vi "SetTriggerCount.vi"(8 "Error In":errorcluster, 10 "Count (1-3000)":u16, 11 "Keithley 6482 In":refnum<visa-resource-name>) -> (0 "Error Out":errorcluster, 3 "Keithley 6482 Out":refnum<visa-resource-name>)   [LabVIEW 8.6, in "Keithley-6482-Visa.lvlib"]
uses:
  Keithley-6482-Visa.lvlib
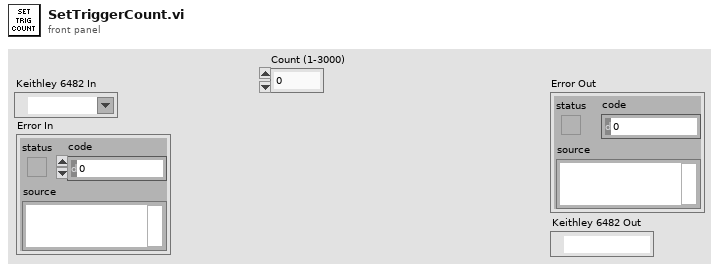
[diagram p1: front panel]
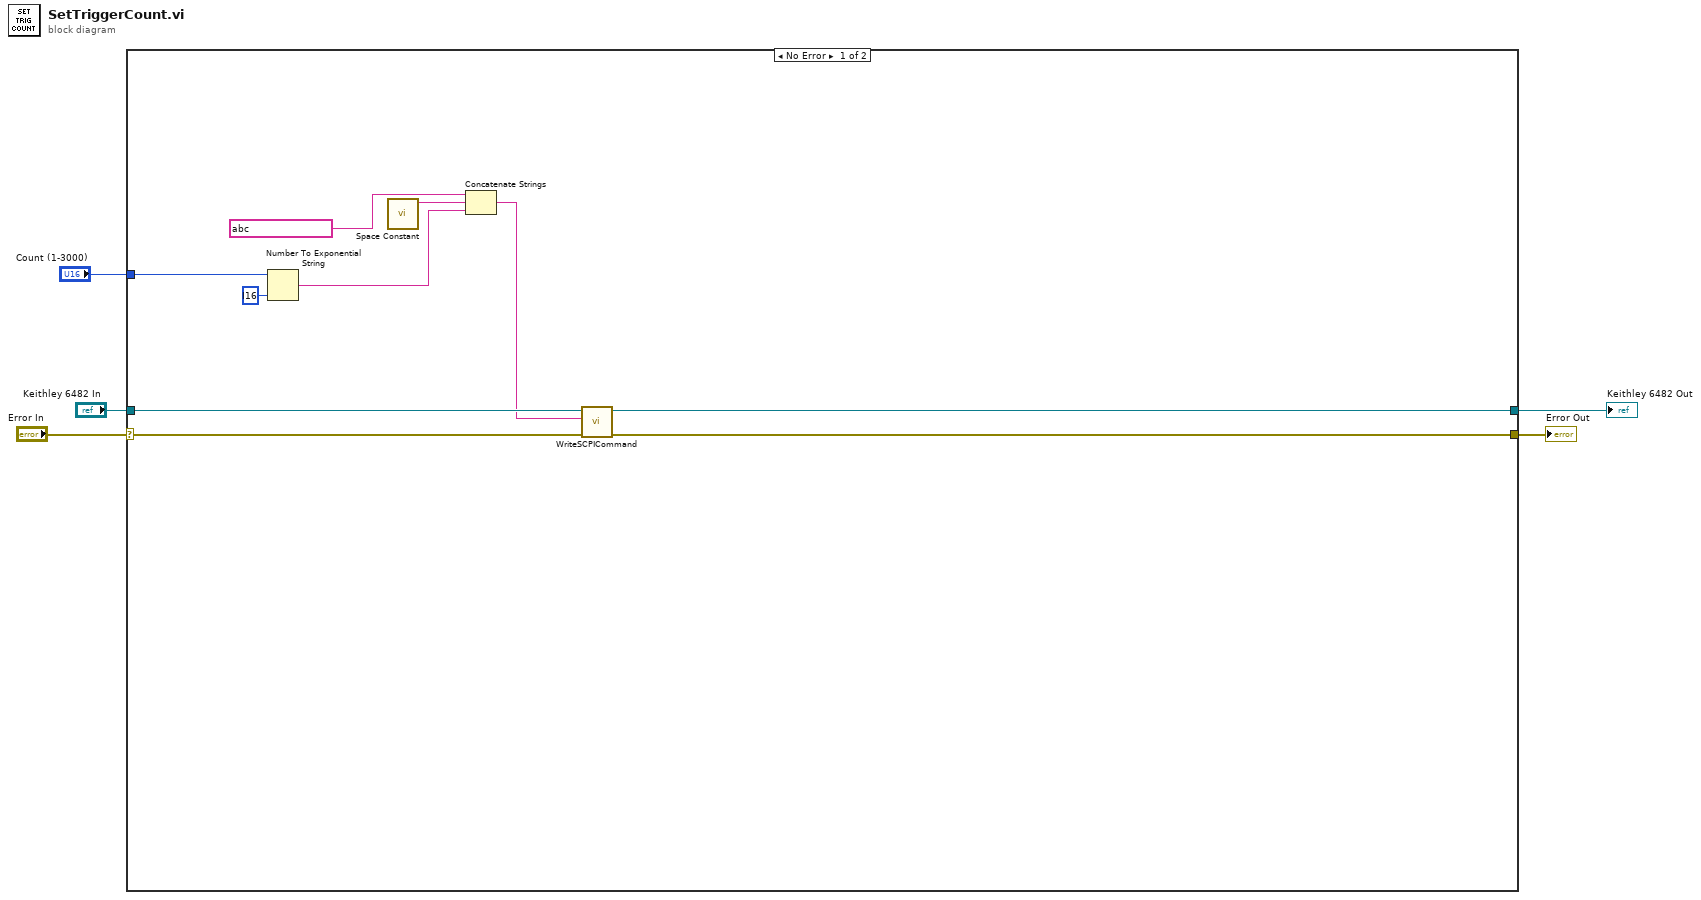
[diagram p0: block diagram]
diagram:
  n1 = case shown="No Error" "Error In" {
    selector: "Error In" -> [w15 w16]
    tunnel: "Keithley 6482 In" -> [w14 w17]
    tunnel: [w7 w16] -> w3
    tunnel: [w8 w17] -> w2
    tunnel: "Count (1-3000)" -> [w11 _]
    frame #0 {
      n2 = Number To Exponential String(number=w11, precision (6)=i16 ?) -> (E-format string=w10:string)  [unwired: 2 in]
      n3 = call <vilib>:"Space Constant.vi"() -> ("String"=w12:string)
      n4 = Concatenate Strings(string ? ("string"), w12, w10) -> (w9:string)
      n5 = call "WriteSCPICommand.vi"("Error In"=w15, "SCPI Command"=w9, "Keithley 6482 In"=w14) -> ("Error Out"=w7:errorcluster, "Keithley 6482 Out"=w8:refnum<visa-resource-name>)  [unwired: 7 in]
    }
    frame #1 {
    }
  }
  "Error Out" <- w3
  "Keithley 6482 Out" <- w2
